vi "Read ADC.vi"(8 "error in (no error)":errorcluster, 10 "Channel":u8, 11 "Simulated Device in":refnum<class "Simulated Device.lvclass">) -> (0 "error out":errorcluster, 1 "Response":string, 2 "ADC Out":u16, 3 "Simulated Device out":refnum<class "Simulated Device.lvclass">)   [LabVIEW 2020, in "Simulated Device.lvclass"]
doc: "Sends \"Read ADC\" command to target device, it returns the value of ADC or an error if target response is invalid or it doesn't respond."
uses:
  Simulated Device.lvclass
  Controls/Device Code.ctl
  Controls/Device Command Code.ctl
  <vilib>/Utility/error.llb/Error Cluster From Error Code.vi
  <vilib>/ErrorRing/Error Ring.xnode
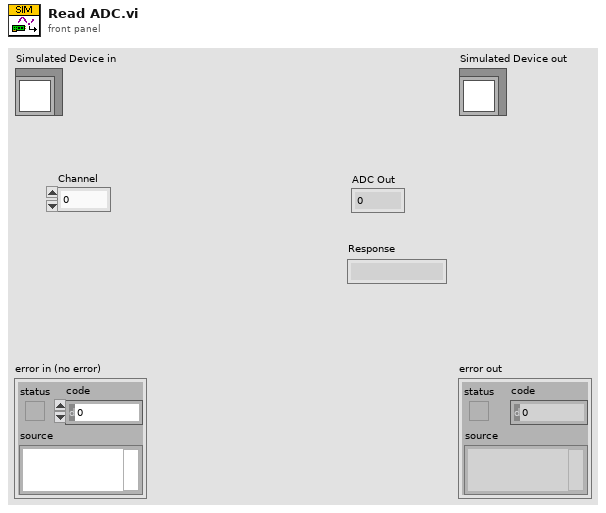
[diagram p1: front panel]
types:
  T1 = typedef "Device Command Code.ctl" = string
  T2 = typedef "Device Code.ctl" = string
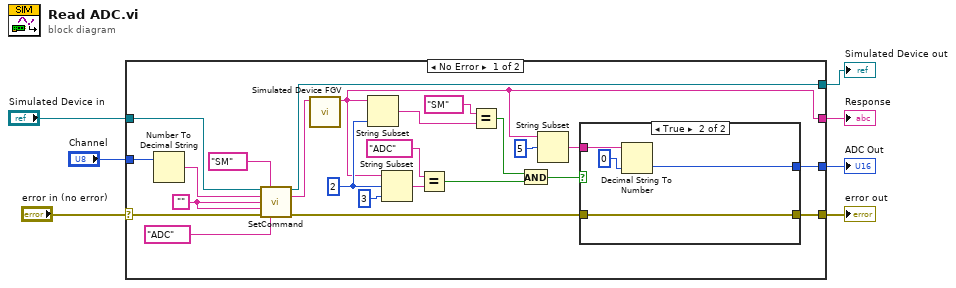
[diagram p0: block diagram]
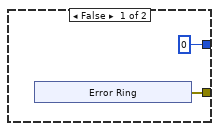
[diagram p2: hidden frame]
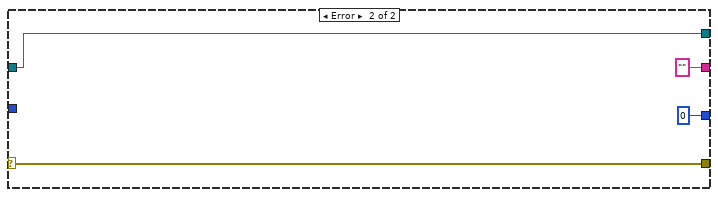
[diagram p3: hidden frame]
diagram:
  n1 = case shown="No Error" "error in (no error)" {
    selector: "error in (no error)" -> [w31 w45]
    tunnel: [w29 w46] -> w5
    tunnel: "Simulated Device in" -> [w30 w46]
    tunnel: [w13 w45] -> w2
    tunnel: "Channel" -> [w12 _]
    tunnel: [w8 "" ("read buffer")] -> w3
    tunnel: [w14 u16 0] -> w4
    frame No Error {
      w25 = 2 ("length (rest)")
      w26 = ""
      n2 = Number To Decimal String(number=w12) -> (decimal integer string=w11:string)  [unwired: 1 in]
      n3 = call-dynamic "SetCommand.vi"("Simulated Device in"=w30, "Device Code"=T2 "SM", "Parameter 1"=w11, "Parameter 2"=w26, "Parameter 3"=w26, "error in (no error)"=w31, "Command Code"=T1 "ADC") -> ("Simulated Device out"=w29:refnum<class "Simulated Device.lvclass">, "Command"=w10:string, "error out"=w9:errorcluster)  [unwired: 6 in]
      n4 = call "Simulated Device FGV.vi"("Request"=w10) -> ("Response"=w8:string)  [unwired: 10 in]
      n5 = String Subset(string=w8, length (rest)=w25) -> (substring=w22:string)  [unwired: 1 in]
      n6 = String Subset(string=w8, offset (0)=w25, length (rest)=3 ("length (rest)")) -> (substring=w20:string)
      n7 = Equal?(x=T1 "ADC" ("Command Code"), y=w20) -> (x = y?=w18:bool)
      n8 = Equal?(x=T2 "SM" ("Device Code"), y=w22) -> (x = y?=w17:bool)
      n9 = And(x=w17, y=w18) -> (x .and. y?=w16:bool)
      n10 = String Subset(string=w8, offset (0)=5) -> (substring=w15:string)  [unwired: 1 in]
      n11 = case shown="True" w16 {
        tunnel: w15 -> [_ w42]
        tunnel: [u16 0 w40] -> w14
        tunnel: [w32 w39] -> w13
        tunnel: w9 -> [_ w39]
        frame False {
          n12 = xnode "Error Ring"() -> ("error out"=w32:errorcluster)
        }
        frame True {
          n13 = Decimal String To Number(string=w42, default (0L)=u16 0 ("default (0 I32)")) -> (number=w40:u16)  [unwired: 1 in, 1 out]
        }
      }
    }
    frame Error {
    }
  }
  "error out" <- w2
  "Simulated Device out" <- w5
  "Response" <- w3
  "ADC Out" <- w4
